vi "EnableChannel.vi"(7 "Channel Name (0: Channel 1)":i32(ring) items=["Channel 1", "Channel 2", "Channel 3", "Channel 4"], 8 "error in (no error)":errorcluster, 10 "Enable":bool, 11 "VISA resource name":refnum<visa-resource-name>) -> (0 "error out":errorcluster, 3 "VISA resource name out":refnum<visa-resource-name>)   [LabVIEW 2023, in "Keysight-DSQx3014T.lvlib"]
doc: "<b>Author:</b> Wolfgang R.\n<b>Description:</b> >>>> Enables the Channel you want >>>"
uses:
  Keysight-DSQx3014T.lvlib
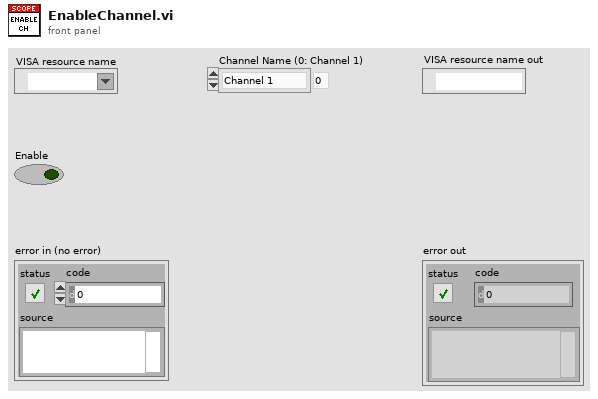
[diagram p1: front panel]
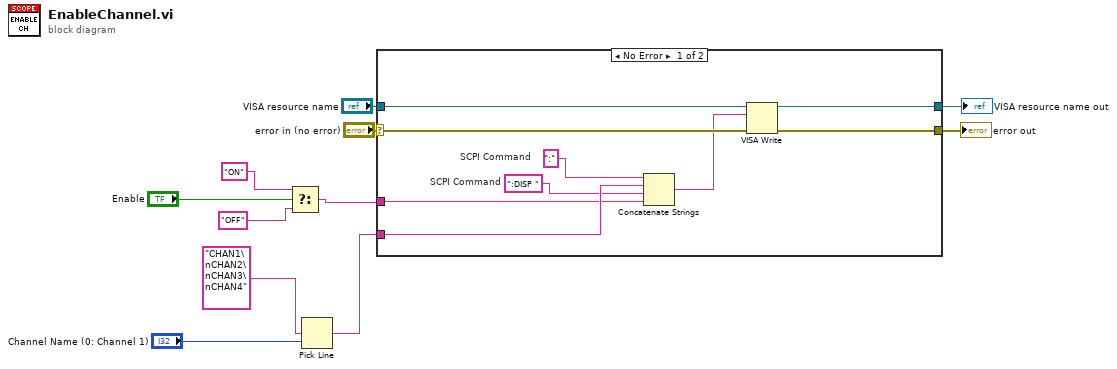
[diagram p0: block diagram]
diagram:
  n1 = Select(t="ON", s="Enable", f="OFF") -> (s? t:f=w4:string)
  n2 = Pick Line(multi-line string="CHAN1\nCHAN2\nCHAN3\nCHAN4", line index="Channel Name (0: Channel 1)") -> (output string=w1:string)  [unwired: 1 out]
  n3 = case shown="No Error" "error in (no error)" {
    selector: "error in (no error)" -> [w17 w22]
    tunnel: [w19 w21] -> w11
    tunnel: [w20 w22] -> w9
    tunnel: "VISA resource name" -> [w18 w21]
    tunnel: w1 -> [w16 _]
    tunnel: w4 -> [w12 _]
    frame No Error {
      w13 = ":DISP "  # SCPI Command
      w14 = ":"  # SCPI Command
      n4 = Concatenate Strings(w14, w16, w13, w12) -> (w15:string)
      n5 = VISA Write(VISA resource name=w18, write buffer=w15, error in (no error)=w17) -> (VISA resource name out=w19:refnum<visa-resource-name>, error out=w20:errorcluster)  [unwired: 1 out]
    }
    frame Error {
    }
  }
  "VISA resource name out" <- w11
  "error out" <- w9
